vi "svc_Compute Scale Factor to Convert V to EU.vi"(10 "pregain [dB]":dbl, 11 "sensor sensitivity [mV/EU]":dbl=1000.0) -> (3 "EU scale factor [EU/V]":dbl=nan format="%_4g")   [LabVIEW 2017]
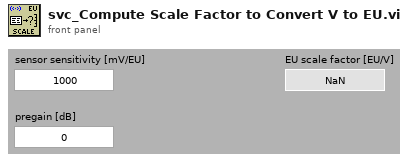
[diagram p1: front panel]
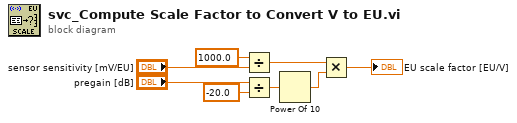
[diagram p0: block diagram]
diagram:
  n1 = Divide(x=1000.0 ("y"), y="sensor sensitivity [mV/EU]") -> (x/y=w4:dbl)
  n2 = Divide(x="pregain [dB]", y=-20.0) -> (x/y=w3:dbl)
  n3 = Power Of 10(x=w3) -> (10^x=w5:dbl)
  n4 = Multiply(x=w4, y=w5) -> (x*y=→"EU scale factor [EU/V]":dbl)
